vi "Configure Spurious Emission (Segment Bandwidth Setup).vi"(0 "VISA resource name":refnum<visa-resource-name>, 5 "Spurious Auto Resolution Bandwidth":i32[](array[ring]) items=["Auto", "Manual"], 7 "Spurious Resolution Bandwidth":i32[](array[ring]) items=["30 Hz", "100 Hz", "300 Hz", "1 kHz", "3 kHz", "10 kHz", "30 kHz", "100 kHz", "300 kHz", "1 MHz", "3 MHz", "50 kHz", "5 MHz", "10 MHz", "20 MHz"], 9 "Spurious Auto Video Bandwidth":i32[](array[ring]) items=["Off", "On"], 11 "error in (no error)":errorcluster, 12 "Spurious Video Bandwidth":i32[](array[ring]) items=["OFF", "1 Hz", "3 Hz", "10 Hz", "30 Hz", "100 Hz", "300 Hz", "1 kHz", "3 kHz", "10 kHz", "30 kHz", "100 kHz", "300 kHz", "1 MHz", "3 MHz", "10 MHz"]) -> (4 "VISA resource name out":refnum<visa-resource-name>, 15 "error out":errorcluster)   [LabVIEW 2020, in "Anritsu Signal Analyzer Series.lvlib"]
doc: "Configures the Bandwidth for segment parameter of Spurious Emission measurement."
uses:
  Anritsu Signal Analyzer Series.lvlib
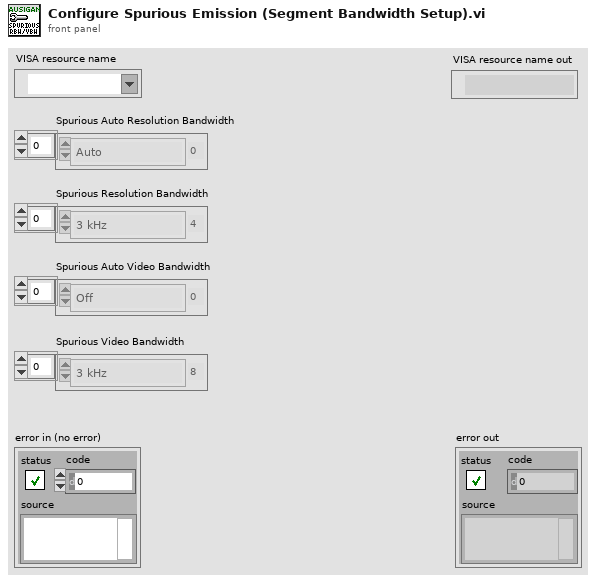
[diagram p1: front panel]
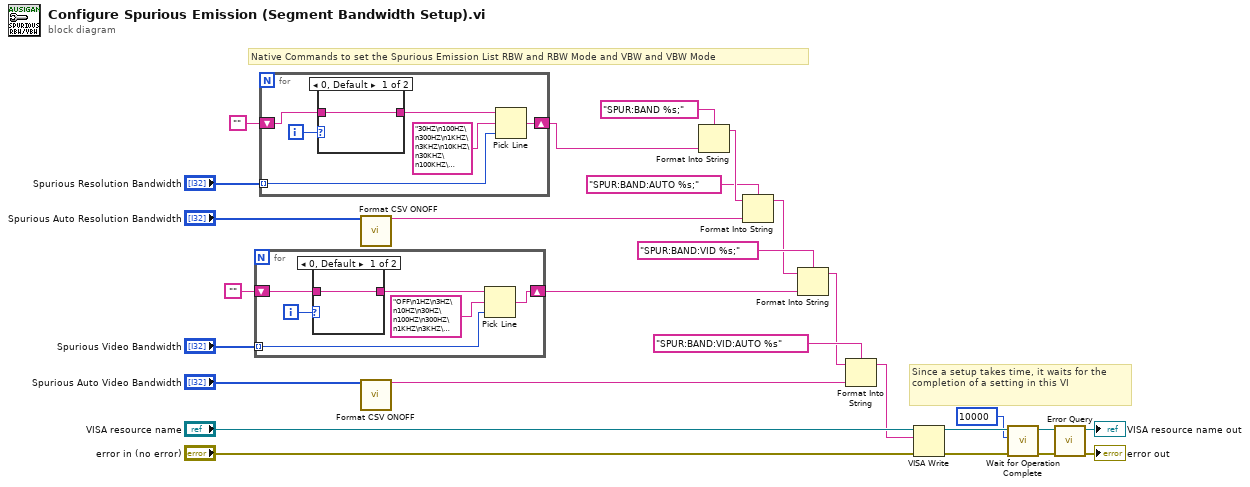
[diagram p0: block diagram]
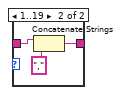
[diagram p2: hidden frame]
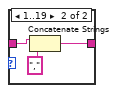
[diagram p3: hidden frame]
diagram:
  # "Since a setup takes time, it waits for the completion of a setting in this VI"
  # "Native Commands to set the Spurious Emission List RBW and RBW Mode and VBW and VBW Mode"
  n1 = for {
    shift-right: [w28] -> w14
    shift-left: "" -> [w32]
    tunnel: "Spurious Video Bandwidth" -> [w30] mode=indexing
    i -> [w33]
    n2 = case shown="0, Default" w33 {
      tunnel: w32 -> [w34 w37]
      tunnel: [w34 w35] -> w29
      frame 0, Default {
      }
      frame 1..19 {
        n3 = Concatenate Strings(w37, "," ("string")) -> (w35:string)
      }
    }
    n4 = Pick Line(string ("")=w29, multi-line string="OFF\n1HZ\n3HZ\n10HZ\n30HZ\n100HZ\n300HZ\n1KHZ\n3KHZ\n10KHZ\n30KHZ\n100KHZ\n300KHZ\n1MHZ\n3MHZ\n5MHZ\n10MHZ\n5KHZ" ("複数行文字列"), line index=w30) -> (output string=w28:string)
  }
  n5 = for {
    shift-right: [w38] -> w20
    shift-left: "" -> [w42]
    tunnel: "Spurious Resolution Bandwidth" -> [w40] mode=indexing
    i -> [w43]
    n6 = case shown="0, Default" w43 {
      tunnel: w42 -> [w44 w47]
      tunnel: [w44 w45] -> w39
      frame 0, Default {
      }
      frame 1..19 {
        n7 = Concatenate Strings(w47, "," ("string")) -> (w45:string)
      }
    }
    n8 = Pick Line(string ("")=w39, multi-line string="30HZ\n100HZ\n300HZ\n1KHZ\n3KHZ\n10KHZ\n30KHZ\n100KHZ\n300KHZ\n1MHZ\n3MHZ\n50KHZ\n5MHZ\n10MHZ\n20MHZ" ("複数行文字列"), line index=w40) -> (output string=w38:string)
  }
  n9 = call "Format CSV ONOFF.vi"("Data_In"="Spurious Auto Resolution Bandwidth") -> ("Data_out"=w5:string)  [unwired: 14 in]
  n10 = call "Format CSV ONOFF.vi"("Data_In"="Spurious Auto Video Bandwidth") -> ("Data_out"=w7:string)  [unwired: 14 in]
  n11 = Format Into String(format string="SPUR:BAND %s;" ("_CommandSet"), w20) -> (resulting string=w18:string)  [unwired: 2 in, 1 out]
  n12 = Format Into String(format string="SPUR:BAND:AUTO %s;" ("_CommandSet"), initial string=w18, w5) -> (resulting string=w12:string)  [unwired: 1 in, 1 out]
  n13 = Format Into String(format string="SPUR:BAND:VID %s;" ("_CommandSet"), initial string=w12, w14) -> (resulting string=w11:string)  [unwired: 1 in, 1 out]
  n14 = Format Into String(format string="SPUR:BAND:VID:AUTO %s" ("_CommandSet"), initial string=w11, w7) -> (resulting string=w10:string)  [unwired: 1 in, 1 out]
  n15 = VISA Write(VISA resource name="VISA resource name", write buffer=w10, error in (no error)="error in (no error)") -> (VISA resource name out=w3:refnum<visa-resource-name>, error out=w2:errorcluster)  [unwired: 1 out]
  n16 = call "Wait for Operation Complete.vi"("error in (no error)"=w2, "Maximum Time (10000mSec)"=10000, "VISA resource name"=w3) -> ("error out"=w8:errorcluster, "VISA resource name out"=w9:refnum<visa-resource-name>)  [unwired: 7 in]
  n17 = call "Error Query.vi"("error in (no error)"=w8, "VISA resource name"=w9) -> ("error out"=→"error out":errorcluster, "VISA resource name out"=→"VISA resource name out":refnum<visa-resource-name>)  [unwired: 6 in, 2 out]
